vi "SoundInput.vi"() -> ()   [LabVIEW 2014]
uses:
  <vilib>/sound2/lvsound2.llb/Sound Data Format.ctl
  <vilib>/sound2/lvsound2.llb/Sampling Mode.ctl
  <vilib>/sound2/lvsound2.llb/Sound Input Read (DBL).vi
panel:
  in  "stop":bool
  out "Waveform Graph":waveform(dbl)[](graph)
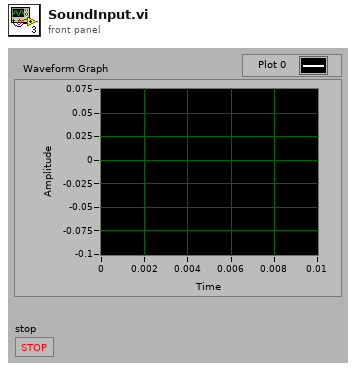
[diagram p1: front panel]
types:
  T1 = typedef "Sampling Mode.ctl" = i32
  T2 = typedef "Sound Data Format.ctl" = cluster{"sample rate (S/s)":dbl, "number of channels":i32, "bits per sample":i32}
  T3 = typedef "Sound Input Task ID.ctl" = u32
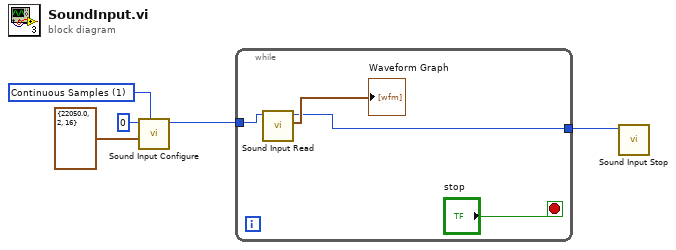
[diagram p0: block diagram]
diagram:
  w2 = T1 1 items=["Finite Samples", "Continuous Samples"] ("sample mode")
  n1 = call <vilib>:"Sound Input Configure.vi"("sample mode"=w2, "sound format"=T2 {"sample rate (S/s)"=22050.0, "number of channels"=2, "bits per sample"=16}, "device ID"=u32 0) -> ("task ID"=w5:T3)  [unwired: 7 in, 1 out]
  n2 = while {
    tunnel: w5 -> [w9]
    tunnel: [w6] -> w1
    stop <- "stop" stop-if-true
    n3 = call-poly <vilib>:"Sound Input Read.vi"("task ID"=w9) -> ("data"=→"Waveform Graph":waveform(dbl)[], "task ID out"=w6:T3)  [unwired: 8 in, 1 out]
  }
  n4 = call <vilib>:"Sound Input Stop.vi"("task ID"=w1) -> ()  [unwired: 9 in, 2 out]
